vi "move_v2.vi"(0 "delay":u32, 2 "Enum":enum16{"hold", "f", "b"}(ring), 3 "D":dbl) -> ()   [LabVIEW 2017]
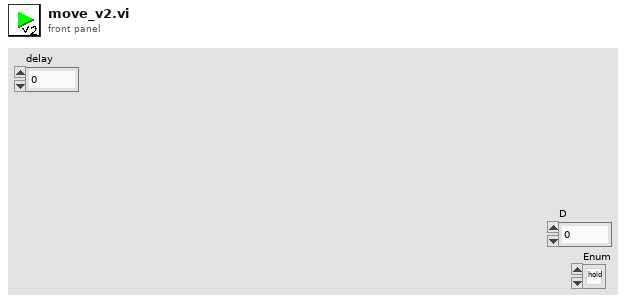
[diagram p1: front panel]
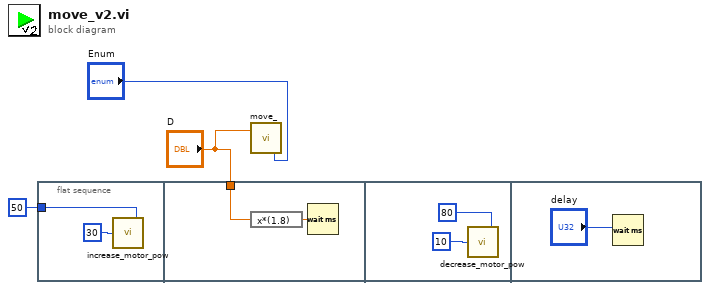
[diagram p0: block diagram]
diagram:
  n1 = flat-sequence {
    tunnel: u32 50 ("delay_per_step") -> [w5]
    tunnel: "D" -> [w6]
    frame #0 {
      n2 = call "increase_motor_pow.vi"("delay_per_step"=w5, "max_pow"=30) -> ()
    }
    frame #1 {
      n3 = expression code="x*(1.8)"(w6) -> (w7:dbl)
      n4 = Wait (ms)(milliseconds to wait=w7) -> ()  [unwired: 1 out]
    }
    frame #2 {
      n5 = call "decrease_motor_pow.vi"("delay_per_step"=80 ("min_pow"), "min_pow"=10) -> ()
    }
    frame #3 {
      n6 = Wait (ms)(milliseconds to wait="delay") -> ()  [unwired: 1 out]
    }
  }
  n7 = call "move_.vi"("Enum"="Enum", "D"="D") -> ()  [unwired: 2 in]
